vi "HEWH Channel Test Labels for RLT.vi"() -> (4 "Station A":T1, 6 "Station B":T1, 8 "Station C":T1, 10 "Station D":T1)   [LabVIEW 2011]
uses:
  Channel Label RLT.ctl
  RLT Stations.ctl
  LabelChannel.ctl
  <vilib>/Utility/file.llb/Write To Spreadsheet File (string).vi
  <vilib>/Utility/file.llb/Read From Spreadsheet File (string).vi
panel:
  out "all rows":string[][](array[string])
  in  "Read":bool
  in  "Write":bool
  in  "Initialize":bool
  in  "Complete":bool
  in  "Panel 3":T3[][](array[typedef])=[[{"Label"="TC Cond1 - IN", "Unit"=enum.""}, {"Label"="TC Cond2", "Unit"=enum.""}, {"Label"="TC Cond3", "Unit"=enum.""}, {"Label"="TC Cond4", "Unit"=enum.""}, {"Label"="TC Cond5", "Unit"=enum.""}, {"Label"="TC Cond6", "Unit"=enum.""}], [{"Label"="TC Cond7", "Unit"=enum.""}, {"Label"="TC Cond8", "Unit"=enum.""}, {"Label"="TC Cond9", "Unit"=enum.""}, {"Label"="TC Cond10", "Unit"=enum.""}, {"Label"="TC Cond11", "Unit"=enum.""}, {"Label"="TC Cond12 - OUT", "Unit"=enum.""}], [{"Label"="TC Xtra 4", "Unit"=enum.""}, {"Label"="TC Xtra 5", "Unit"=enum.""}, {"Label"="TC Xtra 6", "Unit"=enum.""}, {"Label"="TC Xtra 7", "Unit"=enum.""}, {"Label"="TC Xtra 8", "Unit"=enum.""}, {"Label"="TC Xtra 9", "Unit"=enum.""}]]
  in  "Panel 2":T3[][](array[typedef])=[[{"Label"="TC Dry/W bulb 1", "Unit"=enum.""}, {"Label"="TC Dry/W bulb 2", "Unit"=enum.""}, {"Label"="TC Dry/W bulb 3", "Unit"=enum.""}, {"Label"="TC Dry/W bulb 4", "Unit"=enum.""}, {"Label"="TC Tsuction", "Unit"=enum.""}, {"Label"="TC Tdis", "Unit"=enum.""}], [{"Label"="TC Tret", "Unit"=enum.""}, {"Label"="TC Controls 1", "Unit"=enum.""}, {"Label"="TC Controls 2", "Unit"=enum.""}, {"Label"="TC Controls 3", "Unit"=enum.""}, {"Label"="TC Controls 4", "Unit"=enum.""}, {"Label"="TC Controls 5", "Unit"=enum.""}], [{"Label"="TC Shadow T1", "Unit"=enum.""}, {"Label"="TC Shadow T2", "Unit"=enum.""}, {"Label"="TC Shadow T3", "Unit"=enum.""}, {"Label"="TC Shadow T4", "Unit"=enum.""}, {"Label"="TC Shadow T5", "Unit"=enum.""}, {"Label"="TC Shadow T6", "Unit"=enum.""}]]
  in  "Panel 1":T3[][](array[typedef])=[[{"Label"="TC Tree 1 - TOP", "Unit"=enum.""}, {"Label"="TC Tree 2", "Unit"=enum.""}, {"Label"="TC Tree 3", "Unit"=enum.""}, {"Label"="TC Tree 4", "Unit"=enum.""}, {"Label"="TC Tree 5", "Unit"=enum.""}, {"Label"="TC Tree 6 - BOT", "Unit"=enum.""}], [{"Label"="TC Shell 1", "Unit"=enum.""}, {"Label"="TC Shell 2", "Unit"=enum.""}, {"Label"="TC Shell 3", "Unit"=enum.""}, {"Label"="TC Shell 4", "Unit"=enum.""}, {"Label"="TC Evap1 - IN", "Unit"=enum.""}, {"Label"="TC Evap2", "Unit"=enum.""}], [{"Label"="TC Evap3", "Unit"=enum.""}, {"Label"="TC Evap4", "Unit"=enum.""}, {"Label"="TC Evap5 - OUT", "Unit"=enum.""}, {"Label"="TC Xtra 1", "Unit"=enum.""}, {"Label"="TC Xtra 2", "Unit"=enum.""}, {"Label"="TC Xtra 3", "Unit"=enum.""}]]
  in  "Sensor 2":T3
  # "Select Unit (A,B,C,D)  and Add Label. Using the first 10 in Panel 1 is the best."
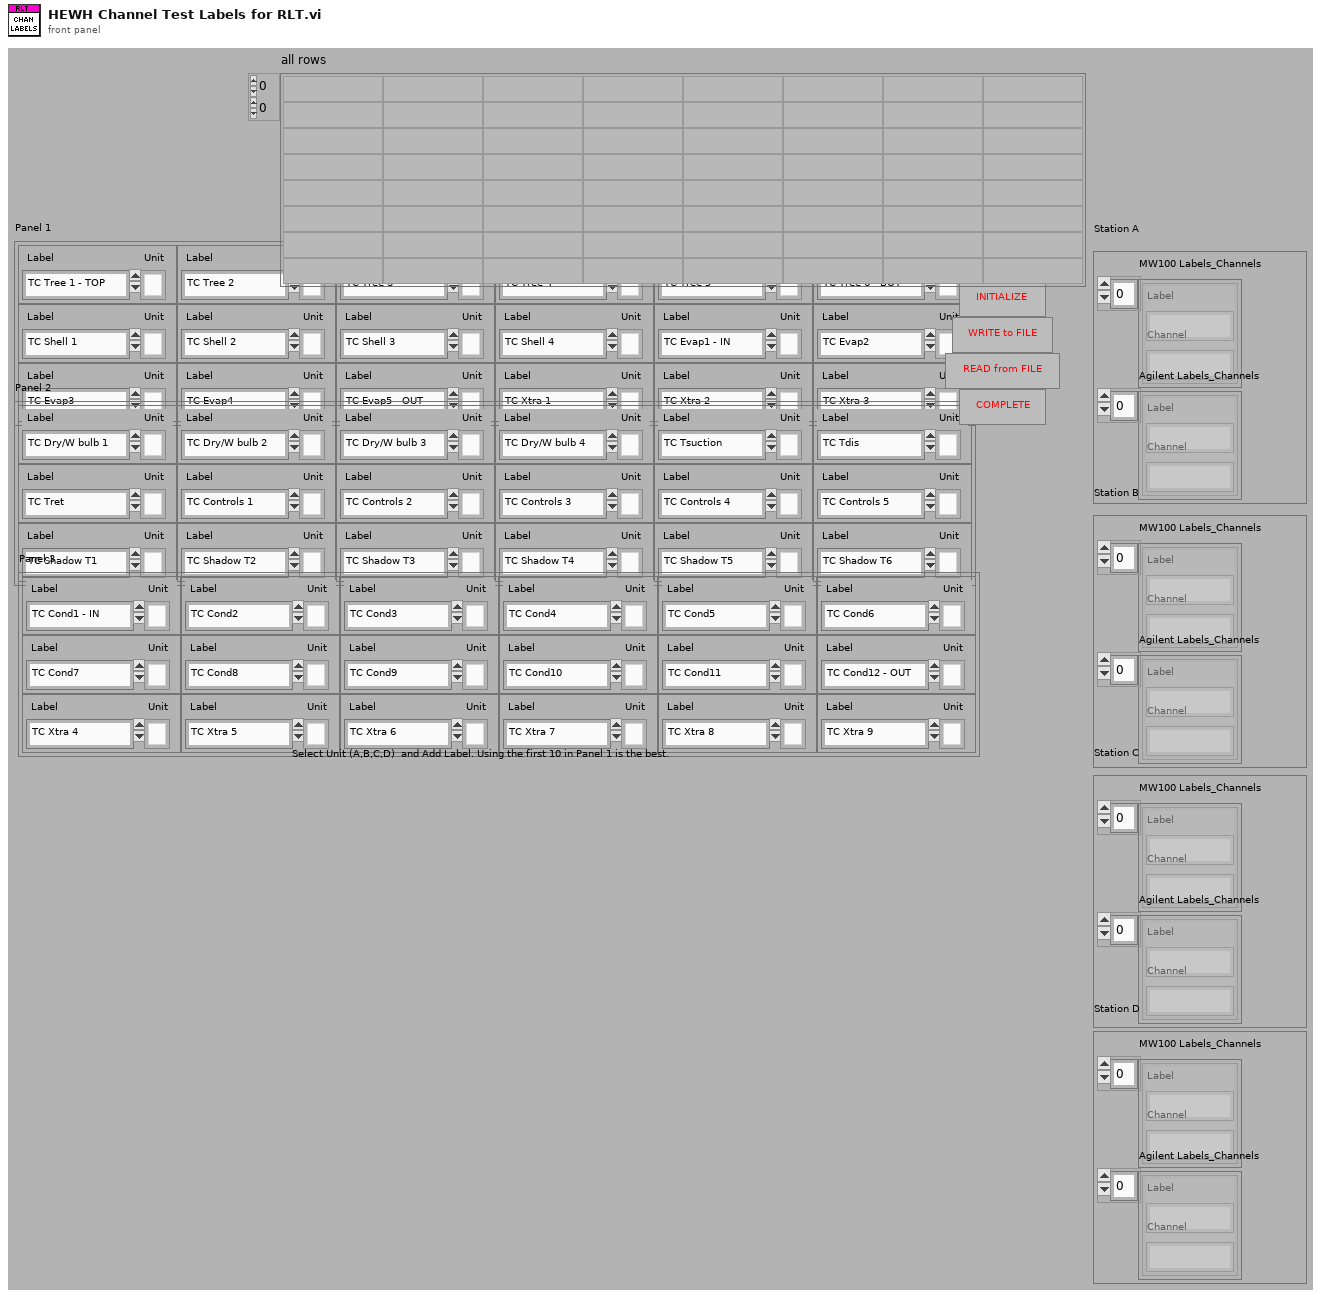
[diagram p1: front panel]
types:
  T1 = typedef "RLT Stations.ctl" = cluster{"MW100 Labels_Channels":T2[], "Agilent Labels_Channels":T2[]}
  T2 = typedef "LabelChannel.ctl" = cluster{"Label":string, "Channel":string}
  T3 = typedef "Channel Label RLT.ctl" = cluster{"Label":string, "Unit":enum16{"", "A", "B", "C", "D"}}
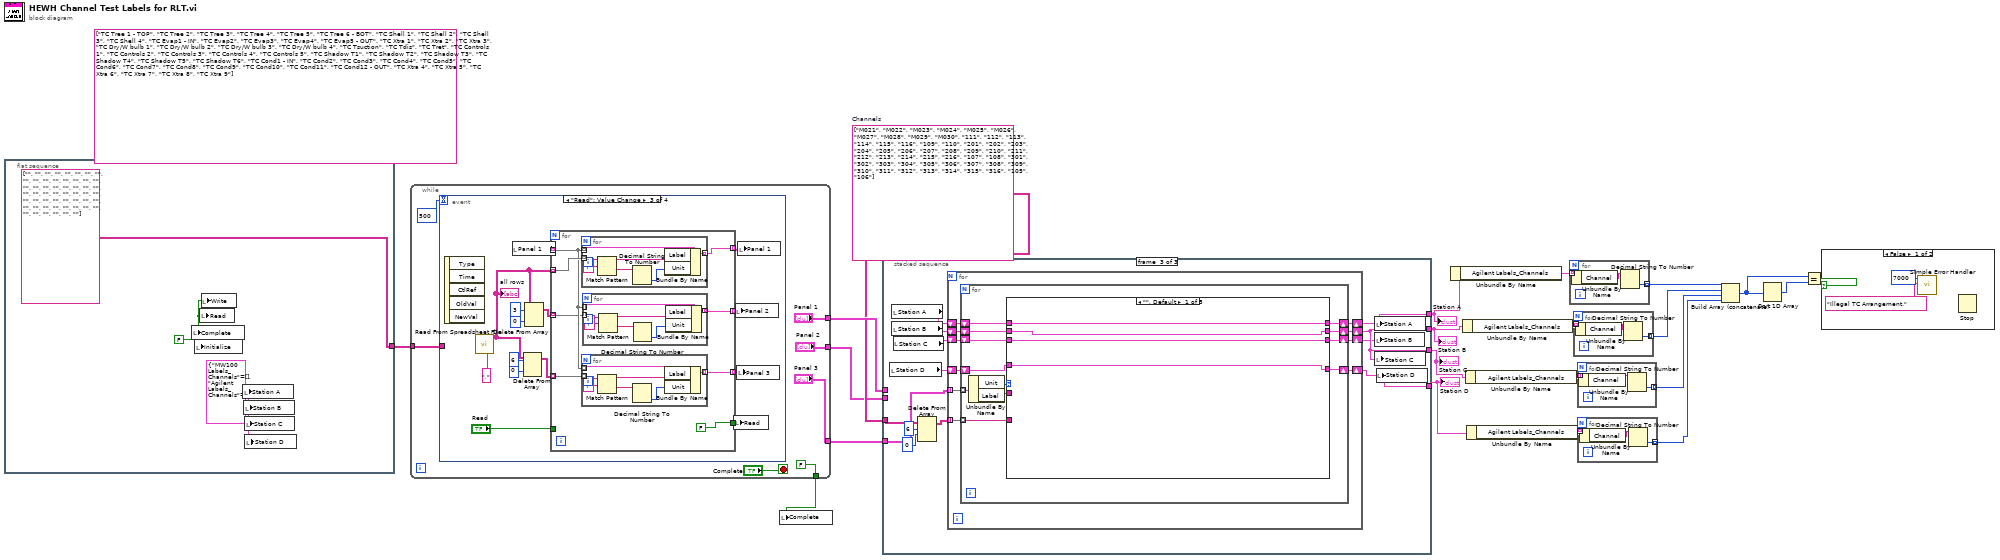
[diagram p0: block diagram]
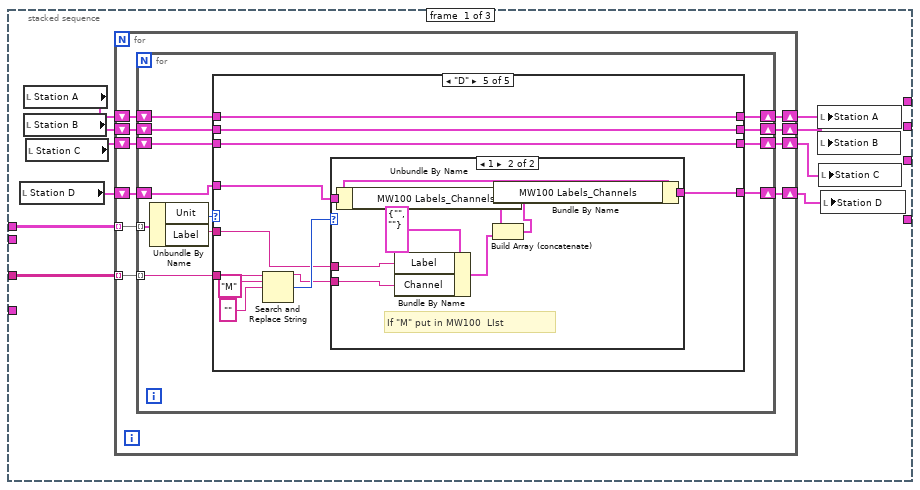
[diagram p3: hidden frame]
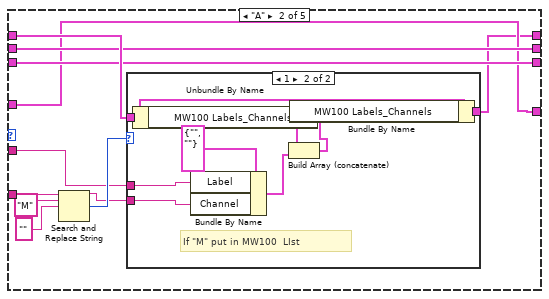
[diagram p5: hidden frame]
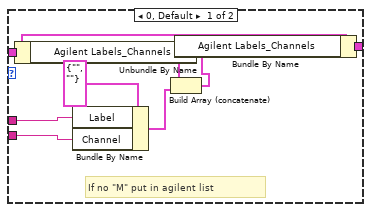
[diagram p6: hidden frame]
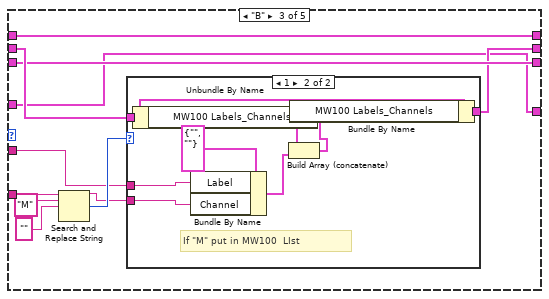
[diagram p7: hidden frame]
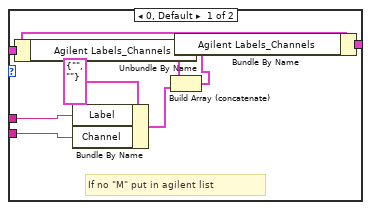
[diagram p8: hidden frame]
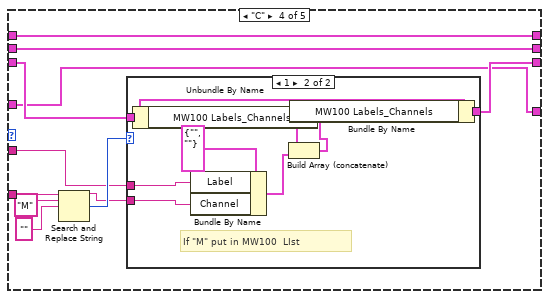
[diagram p9: hidden frame]
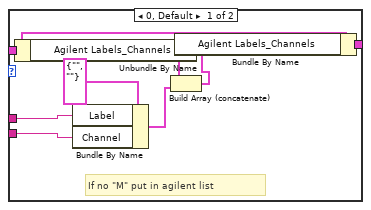
[diagram p10: hidden frame]
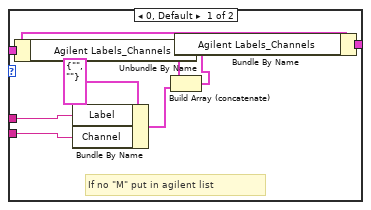
[diagram p11: hidden frame]
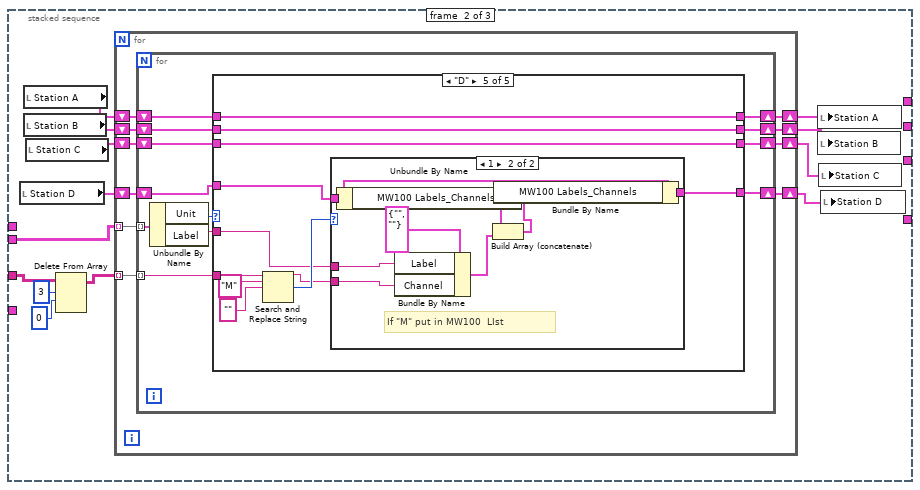
[diagram p12: hidden frame]
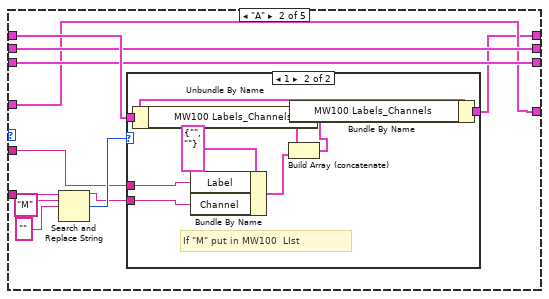
[diagram p14: hidden frame]
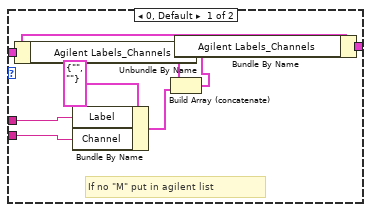
[diagram p15: hidden frame]
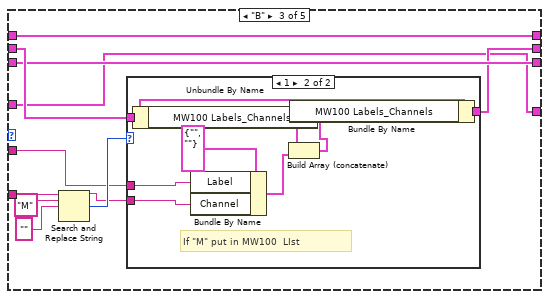
[diagram p16: hidden frame]
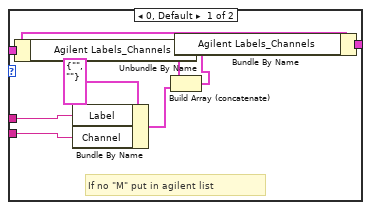
[diagram p17: hidden frame]
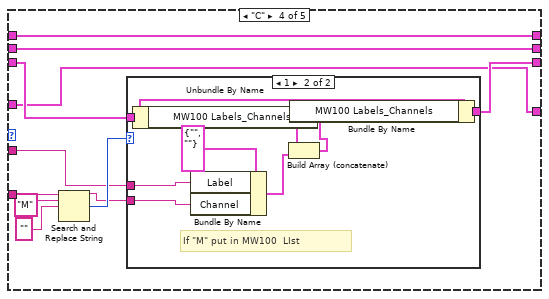
[diagram p18: hidden frame]
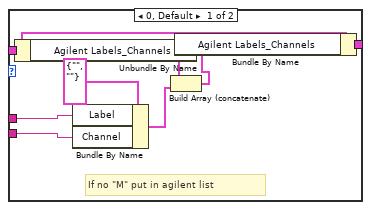
[diagram p19: hidden frame]
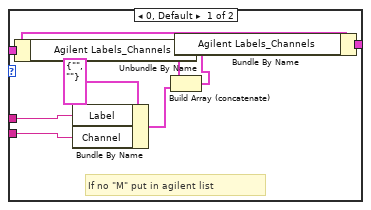
[diagram p20: hidden frame]
diagram:
  (unwired) string[][] [["TC Tree 1 - TOP", "TC Tree 2", "TC Tree 3", "TC Tree 4", "TC Tree 5", "TC Tree 6 - BOT"], ["TC Shell 1", "TC Shell 2", "TC Shell 3", "TC Shell 4", "TC Evap1 - IN", "TC Evap2"], ["TC Evap3", "TC Evap4", "TC Evap5 - OUT", "TC Xtra 1", "TC Xtra 2", "TC Xtra 3"], ["TC Dry/W bulb 1", "TC Dry/W bulb 2", "TC Dry/W bulb 3", "TC Dry/W bulb 4", "TC Tsuction", "TC Tdis"], ["TC Tret", "TC Controls 1", "TC Controls 2", "TC Controls 3", "TC Controls 4", "TC Controls 5"], ["TC Shadow T1", "TC Shadow T2", "TC Shadow T3", "TC Shadow T4", "TC Shadow T5", "TC Shadow T6"], ["TC Cond1 - IN", "TC Cond2", "TC Cond3", "TC Cond4", "TC Cond5", "TC Cond6"], ["TC Cond7", "TC Cond8", "TC Cond9", "TC Cond10", "TC Cond11", "TC Cond12 - OUT"], ["TC Xtra 4", "TC Xtra 5", "TC Xtra 6", "TC Xtra 7", "TC Xtra 8", "TC Xtra 9"]] ("Array")
  w18 = string[][] [["M021", "M022", "M023", "M024", "M025", "M026"], ["M027", "M028", "M029", "M030", "111", "112"], ["113", "114", "115", "116", "109", "110"], ["201", "202", "203", "204", "205", "206"], ["207", "208", "209", "210", "211", "212"], ["213", "214", "215", "216", "107", "108"], ["301", "302", "303", "304", "305", "306"], ["307", "308", "309", "310", "311", "312"], ["313", "314", "315", "316", "105", "106"]]  # Channels
  n1 = flat-sequence {
    tunnel: [string[][] [["", "", "", "", "", ""], ["", "", "", "", "", ""], ["", "", "", "", "", ""], ["", "", "", "", "", ""], ["", "", "", "", "", ""], ["", "", "", "", "", ""], ["", "", "", "", "", ""], ["", "", "", "", "", ""], ["", "", "", "", "", ""]] ("Array")] -> w21
    frame #0 {
      w24 = T1 {"MW100 Labels_Channels"=[], "Agilent Labels_Channels"=[]} ("Station A")
      w22 = FALSE ("Read None")
      n2 = local write "Complete"(w22) -> ()
      n3 = local write "Initialize"(w22) -> ()
      n4 = local write "Read"(w22) -> ()
      n5 = local write "Write"(w22) -> ()
      n6 = local write "Station A"(w24) -> ()
      n7 = local write "Station B"(w24) -> ()
      n8 = local write "Station C"(w24) -> ()
      n9 = local write "Station D"(w24) -> ()
    }
  }
  n10 = while {
    tunnel: w21 -> [w31]
    tunnel: ["Panel 1"] -> w19
    tunnel: ["Panel 2"] -> w17
    tunnel: ["Panel 3"] -> w16
    tunnel: [FALSE ("Read None")] -> w20
    stop <- "Complete" stop-if-true
    n11 = event shown="[2] \"Read\": Value Change" {
      selector: _ -> [_ _ _ _]
      dyn-events: _ -> [_ _ _ _]
      timeout: 500 -> [_ _ _ _]
      tunnel: w31 -> [w42 _ _ _]
      event "Initialize": Value Change {
        n12 = event-data() -> ()  [unwired: 1 in, 5 out]
        n13 = for {
          tunnel: [w45] -> w41 mode=indexing
          tunnel: w42 -> [w44] mode=indexing
          tunnel: [FALSE ("Read None")] -> w32
          n14 = for {
            tunnel: [w49] -> w45 mode=indexing
            tunnel: w44 -> [w48] mode=indexing
            n15 = Bundle By Name(cluster="Sensor 2", "Label"=w48, "Unit"=enum16{"", "A", "B", "C", "D"}."") -> (w49:T3)
          }
        }
        n16 = Delete From Array(array=w41, length=3, index (row)=0) -> (deleted portion=w35:T3[][], array with subset deleted=w36:T3[][])  [unwired: 1 in]
        n17 = local write "Initialize"(w32) -> ()
        n18 = local write "Panel 1"(w35) -> ()
        n19 = Delete From Array(array=w36, length=3, index (row)=0) -> (deleted portion=w34:T3[][], array with subset deleted=w33:T3[][])  [unwired: 1 in]
        n20 = local write "Panel 2"(w34) -> ()
        n21 = local write "Panel 3"(w33) -> ()
      }
      event "Write": Value Change {
        n22 = event-data() -> ()  [unwired: 1 in, 5 out]
        n23 = local read "Panel 3"() -> (w57:T3[][])
        n24 = local read "Panel 2"() -> (w58:T3[][])
        n25 = local read "Panel 1"() -> (w59:T3[][])
        n26 = for {
          tunnel: w59 -> [w78] mode=indexing
          tunnel: [w77] -> w54 mode=indexing
          tunnel: "Write" -> [_]
          tunnel: [FALSE ("Read")] -> w50
          n27 = for {
            tunnel: w78 -> [w84] mode=indexing
            tunnel: [w79] -> w77 mode=indexing
            n28 = Unbundle By Name(w84) -> ("Label"=w82:string, "Unit"=w83:enum16{"", "A", "B", "C", "D"})
            n29 = Number To Decimal String(number=w83) -> (decimal integer string=w80:string)  [unwired: 1 in]
            n30 = Concatenate Strings(w82, "/" ("string"), w80) -> (w79:string)
          }
        }
        n31 = for {
          tunnel: w58 -> [w69] mode=indexing
          tunnel: [w68] -> w55 mode=indexing
          n32 = for {
            tunnel: w69 -> [w75] mode=indexing
            tunnel: [w70] -> w68 mode=indexing
            n33 = Unbundle By Name(w75) -> ("Label"=w73:string, "Unit"=w74:enum16{"", "A", "B", "C", "D"})
            n34 = Number To Decimal String(number=w74) -> (decimal integer string=w71:string)  [unwired: 1 in]
            n35 = Concatenate Strings(w73, "/" ("string"), w71) -> (w70:string)
          }
        }
        n36 = for {
          tunnel: w57 -> [w61] mode=indexing
          tunnel: [w60] -> w56 mode=indexing
          n37 = for {
            tunnel: w61 -> [w67] mode=indexing
            tunnel: [w62] -> w60 mode=indexing
            n38 = Unbundle By Name(w67) -> ("Label"=w65:string, "Unit"=w66:enum16{"", "A", "B", "C", "D"})
            n39 = Number To Decimal String(number=w66) -> (decimal integer string=w63:string)  [unwired: 1 in]
            n40 = Concatenate Strings(w65, "/" ("string"), w63) -> (w62:string)
          }
        }
        n41 = Build Array (concatenate)(w54, w55, w56) -> (w53:string[][])
        n42 = local write "Write"(w50) -> ()
        n43 = call-poly <vilib>:"Write To Spreadsheet File.vi"("delimiter (\\t)"="," ("delimiter (\\t)"), "2D data"=w53) -> ()  [unwired: 6 in, 1 out]
      }
      event "Read": Value Change {
        n44 = event-data() -> ()  [unwired: 1 in, 5 out]
        n45 = call-poly <vilib>:"Read From Spreadsheet File.vi"("delimiter (\\t)"="," ("delimiter (\\t)")) -> ("all rows"=w90:string[][])  [unwired: 6 in, 4 out]
        "all rows" <- w90
        n46 = local read "Panel 1"() -> (w97:T3[][])
        n47 = Delete From Array(array=w90, length=6, index (row)=0) -> (array with subset deleted=w89:string[][])  [unwired: 1 in, 1 out]
        n48 = Delete From Array(array=w90, length=3, index (row)=0) -> (array with subset deleted=w93:string[][])  [unwired: 1 in, 1 out]
        n49 = for {
          tunnel: w97 -> [w104] mode=indexing
          tunnel: w90 -> [w106] mode=indexing
          tunnel: [w105] -> w96 mode=indexing
          tunnel: w93 -> [w103] mode=indexing
          tunnel: w89 -> [w102] mode=indexing
          tunnel: [w101] -> w88 mode=indexing
          tunnel: [w100] -> w87 mode=indexing
          tunnel: "Read" -> [_]
          tunnel: [FALSE ("Read")] -> w85
          n50 = for {
            tunnel: w104 -> [w125] mode=indexing
            tunnel: w106 -> [w127] mode=indexing
            tunnel: [w122] -> w105 mode=indexing
            n51 = Match Pattern(string=w127, regular expression="/") -> (before substring=w124:string, after substring=w123:string)  [unwired: 1 in, 2 out]
            n52 = Decimal String To Number(string=w123) -> (number=w121:i32)  [unwired: 2 in, 1 out]
            n53 = Bundle By Name(cluster=w125, "Label"=w124, "Unit"=w121) -> (w122:T3)
          }
          n54 = for {
            tunnel: w104 -> [w111] mode=indexing
            tunnel: w102 -> [w113] mode=indexing
            tunnel: [w108] -> w100 mode=indexing
            n55 = Match Pattern(string=w113, regular expression="/") -> (before substring=w110:string, after substring=w109:string)  [unwired: 1 in, 2 out]
            n56 = Decimal String To Number(string=w109) -> (number=w107:i32)  [unwired: 2 in, 1 out]
            n57 = Bundle By Name(cluster=w111, "Label"=w110, "Unit"=w107) -> (w108:T3)
          }
          n58 = for {
            tunnel: w104 -> [w118] mode=indexing
            tunnel: w103 -> [w120] mode=indexing
            tunnel: [w115] -> w101 mode=indexing
            n59 = Match Pattern(string=w120, regular expression="/") -> (before substring=w117:string, after substring=w116:string)  [unwired: 1 in, 2 out]
            n60 = Decimal String To Number(string=w116) -> (number=w114:i32)  [unwired: 2 in, 1 out]
            n61 = Bundle By Name(cluster=w118, "Label"=w117, "Unit"=w114) -> (w115:T3)
          }
        }
        n62 = local write "Read"(w85) -> ()
        n63 = local write "Panel 2"(w88) -> ()
        n64 = local write "Panel 3"(w87) -> ()
        n65 = local write "Panel 1"(w96) -> ()
      }
      event Timeout {
        n66 = event-data() -> ()  [unwired: 1 in, 2 out]
      }
    }
  }
  n67 = local write "Complete"(w20) -> ()
  n68 = stacked-sequence {
    tunnel: w19 -> [w137 _ _]
    tunnel: w18 -> [w136 w275 w419]
    tunnel: w17 -> [_ w276 _]
    tunnel: w16 -> [_ _ w427]
    tunnel: [_ _ w426] -> w8
    tunnel: [_ _ w425] -> w9
    tunnel: [_ _ w424] -> w13
    tunnel: [_ _ w423] -> w15
    frame #0 {
      n69 = local read "Station D"() -> (w128:T1)
      n70 = local read "Station A"() -> (w131:T1)
      n71 = local read "Station B"() -> (w130:T1)
      n72 = local read "Station C"() -> (w129:T1)
      n73 = for {
        tunnel: w137 -> [w147] mode=indexing
        tunnel: w136 -> [w145] mode=indexing
        shift-right: [w144] -> w135
        shift-left: w131 -> [w146]
        shift-right: [w142] -> w134
        shift-left: w130 -> [w143]
        shift-right: [w140] -> w133
        shift-left: w129 -> [w141]
        shift-right: [w138] -> w132
        shift-left: w128 -> [w139]
        n74 = for {
          tunnel: w147 -> [w159] mode=indexing
          tunnel: w145 -> [w157] mode=indexing
          shift-right: [w148] -> w144
          shift-left: w146 -> [w153]
          shift-right: [w152] -> w142
          shift-left: w143 -> [w151]
          shift-right: [w150] -> w140
          shift-left: w141 -> [w149]
          shift-right: [w154] -> w138
          shift-left: w139 -> [w155]
          n75 = Unbundle By Name(w159) -> ("Unit"=w158:enum16{"", "A", "B", "C", "D"}, "Label"=w156:string)
          n76 = case shown="\"D\"" w158 {
            tunnel: w155 -> [w160 w165 w191 w218 w251]
            tunnel: w157 -> [_ w174 w201 w228 w255]
            tunnel: w156 -> [_ w169 w196 w223 w249]
            tunnel: [w160 w165 w191 w218 w248] -> w154
            tunnel: w153 -> [w163 w168 w195 w222 w247]
            tunnel: [w162 w167 w192 w221 w246] -> w152
            tunnel: w151 -> [w162 w167 w194 w221 w246]
            tunnel: [w161 w166 w193 w219 w245] -> w150
            tunnel: w149 -> [w161 w166 w193 w220 w245]
            tunnel: [w163 w164 w195 w222 w247] -> w148
            frame "", Default {
            }
            frame "A" {
              n77 = Search and Replace String(input string=w174, search string="M", replace string="" ("replace string (\"\")")) -> (result string=w170:string, number of replacements=w171:i32)  [unwired: 5 in, 2 out]
              n78 = case shown="1" w171 {
                tunnel: w168 -> [w176 w184]
                tunnel: w170 -> [w180 w188]
                tunnel: w169 -> [w179 w187]
                tunnel: [w175 w183] -> w164
                frame 0, Default {
                  # "If no \"M\" put in agilent list"
                  n79 = Unbundle By Name(w176) -> ("Agilent Labels_Channels"=w182:T2[])
                  n80 = Bundle By Name(cluster=T2 {"Label"="", "Channel"=""} ("input cluster"), "Label"=w179, "Channel"=w180) -> (w178:T2)
                  n81 = Build Array (concatenate)(w182, w178) -> (w177:T2[])
                  n82 = Bundle By Name(cluster=w176, "Agilent Labels_Channels"=w177) -> (w175:T1)
                }
                frame 1 {
                  # "If \"M\" put in MW100  LIst"
                  n83 = Unbundle By Name(w184) -> ("MW100 Labels_Channels"=w190:T2[])
                  n84 = Bundle By Name(cluster=T2 {"Label"="", "Channel"=""} ("input cluster"), "Label"=w187, "Channel"=w188) -> (w186:T2)
                  n85 = Build Array (concatenate)(w190, w186) -> (w185:T2[])
                  n86 = Bundle By Name(cluster=w184, "MW100 Labels_Channels"=w185) -> (w183:T1)
                }
              }
            }
            frame "B" {
              n87 = Search and Replace String(input string=w201, search string="M", replace string="" ("replace string (\"\")")) -> (result string=w197:string, number of replacements=w198:i32)  [unwired: 5 in, 2 out]
              n88 = case shown="1" w198 {
                tunnel: w194 -> [w203 w211]
                tunnel: w197 -> [w207 w215]
                tunnel: w196 -> [w206 w214]
                tunnel: [w202 w210] -> w192
                frame 0, Default {
                  # "If no \"M\" put in agilent list"
                  n89 = Unbundle By Name(w203) -> ("Agilent Labels_Channels"=w209:T2[])
                  n90 = Bundle By Name(cluster=T2 {"Label"="", "Channel"=""} ("input cluster"), "Label"=w206, "Channel"=w207) -> (w205:T2)
                  n91 = Build Array (concatenate)(w209, w205) -> (w204:T2[])
                  n92 = Bundle By Name(cluster=w203, "Agilent Labels_Channels"=w204) -> (w202:T1)
                }
                frame 1 {
                  # "If \"M\" put in MW100  LIst"
                  n93 = Unbundle By Name(w211) -> ("MW100 Labels_Channels"=w217:T2[])
                  n94 = Bundle By Name(cluster=T2 {"Label"="", "Channel"=""} ("input cluster"), "Label"=w214, "Channel"=w215) -> (w213:T2)
                  n95 = Build Array (concatenate)(w217, w213) -> (w212:T2[])
                  n96 = Bundle By Name(cluster=w211, "MW100 Labels_Channels"=w212) -> (w210:T1)
                }
              }
            }
            frame "C" {
              n97 = Search and Replace String(input string=w228, search string="M", replace string="" ("replace string (\"\")")) -> (result string=w224:string, number of replacements=w225:i32)  [unwired: 5 in, 2 out]
              n98 = case shown="1" w225 {
                tunnel: w220 -> [w230 w238]
                tunnel: w224 -> [w234 w242]
                tunnel: w223 -> [w233 w241]
                tunnel: [w229 w237] -> w219
                frame 0, Default {
                  # "If no \"M\" put in agilent list"
                  n99 = Unbundle By Name(w230) -> ("Agilent Labels_Channels"=w236:T2[])
                  n100 = Bundle By Name(cluster=T2 {"Label"="", "Channel"=""} ("input cluster"), "Label"=w233, "Channel"=w234) -> (w232:T2)
                  n101 = Build Array (concatenate)(w236, w232) -> (w231:T2[])
                  n102 = Bundle By Name(cluster=w230, "Agilent Labels_Channels"=w231) -> (w229:T1)
                }
                frame 1 {
                  # "If \"M\" put in MW100  LIst"
                  n103 = Unbundle By Name(w238) -> ("MW100 Labels_Channels"=w244:T2[])
                  n104 = Bundle By Name(cluster=T2 {"Label"="", "Channel"=""} ("input cluster"), "Label"=w241, "Channel"=w242) -> (w240:T2)
                  n105 = Build Array (concatenate)(w244, w240) -> (w239:T2[])
                  n106 = Bundle By Name(cluster=w238, "MW100 Labels_Channels"=w239) -> (w237:T1)
                }
              }
            }
            frame "D" {
              n107 = Search and Replace String(input string=w255, search string="M", replace string="" ("replace string (\"\")")) -> (result string=w250:string, number of replacements=w252:i32)  [unwired: 5 in, 2 out]
              n108 = case shown="1" w252 {
                tunnel: w251 -> [w257 w265]
                tunnel: w250 -> [w261 w269]
                tunnel: w249 -> [w260 w268]
                tunnel: [w256 w264] -> w248
                frame 0, Default {
                  # "If no \"M\" put in agilent list"
                  n109 = Unbundle By Name(w257) -> ("Agilent Labels_Channels"=w263:T2[])
                  n110 = Bundle By Name(cluster=T2 {"Label"="", "Channel"=""} ("input cluster"), "Label"=w260, "Channel"=w261) -> (w259:T2)
                  n111 = Build Array (concatenate)(w263, w259) -> (w258:T2[])
                  n112 = Bundle By Name(cluster=w257, "Agilent Labels_Channels"=w258) -> (w256:T1)
                }
                frame 1 {
                  # "If \"M\" put in MW100  LIst"
                  n113 = Unbundle By Name(w265) -> ("MW100 Labels_Channels"=w271:T2[])
                  n114 = Bundle By Name(cluster=T2 {"Label"="", "Channel"=""} ("input cluster"), "Label"=w268, "Channel"=w269) -> (w267:T2)
                  n115 = Build Array (concatenate)(w271, w267) -> (w266:T2[])
                  n116 = Bundle By Name(cluster=w265, "MW100 Labels_Channels"=w266) -> (w264:T1)
                }
              }
            }
          }
        }
      }
      n117 = local write "Station A"(w135) -> ()
      n118 = local write "Station B"(w134) -> ()
      n119 = local write "Station C"(w133) -> ()
      n120 = local write "Station D"(w132) -> ()
    }
    frame #1 {
      n121 = local read "Station D"() -> (w277:T1)
      n122 = local read "Station A"() -> (w280:T1)
      n123 = local read "Station B"() -> (w279:T1)
      n124 = local read "Station C"() -> (w278:T1)
      n125 = Delete From Array(array=w275, length=3, index (row)=0) -> (array with subset deleted=w272:string[][])  [unwired: 1 in, 1 out]
      n126 = for {
        tunnel: w276 -> [w294] mode=indexing
        tunnel: w272 -> [w292] mode=indexing
        shift-right: [w291] -> w284
        shift-left: w280 -> [w293]
        shift-right: [w289] -> w283
        shift-left: w279 -> [w290]
        shift-right: [w287] -> w282
        shift-left: w278 -> [w288]
        shift-right: [w285] -> w281
        shift-left: w277 -> [w286]
        n127 = for {
          tunnel: w294 -> [w306] mode=indexing
          tunnel: w292 -> [w304] mode=indexing
          shift-right: [w295] -> w291
          shift-left: w293 -> [w300]
          shift-right: [w299] -> w289
          shift-left: w290 -> [w298]
          shift-right: [w297] -> w287
          shift-left: w288 -> [w296]
          shift-right: [w301] -> w285
          shift-left: w286 -> [w302]
          n128 = Unbundle By Name(w306) -> ("Unit"=w305:enum16{"", "A", "B", "C", "D"}, "Label"=w303:string)
          n129 = case shown="\"D\"" w305 {
            tunnel: w302 -> [w307 w312 w338 w365 w398]
            tunnel: w304 -> [_ w321 w348 w375 w402]
            tunnel: w303 -> [_ w316 w343 w370 w396]
            tunnel: [w307 w312 w338 w365 w395] -> w301
            tunnel: w300 -> [w310 w315 w342 w369 w394]
            tunnel: [w309 w314 w339 w368 w393] -> w299
            tunnel: w298 -> [w309 w314 w341 w368 w393]
            tunnel: [w308 w313 w340 w366 w392] -> w297
            tunnel: w296 -> [w308 w313 w340 w367 w392]
            tunnel: [w310 w311 w342 w369 w394] -> w295
            frame "", Default {
            }
            frame "A" {
              n130 = Search and Replace String(input string=w321, search string="M", replace string="" ("replace string (\"\")")) -> (result string=w317:string, number of replacements=w318:i32)  [unwired: 5 in, 2 out]
              n131 = case shown="1" w318 {
                tunnel: w315 -> [w323 w331]
                tunnel: w317 -> [w327 w335]
                tunnel: w316 -> [w326 w334]
                tunnel: [w322 w330] -> w311
                frame 0, Default {
                  # "If no \"M\" put in agilent list"
                  n132 = Unbundle By Name(w323) -> ("Agilent Labels_Channels"=w329:T2[])
                  n133 = Bundle By Name(cluster=T2 {"Label"="", "Channel"=""} ("input cluster"), "Label"=w326, "Channel"=w327) -> (w325:T2)
                  n134 = Build Array (concatenate)(w329, w325) -> (w324:T2[])
                  n135 = Bundle By Name(cluster=w323, "Agilent Labels_Channels"=w324) -> (w322:T1)
                }
                frame 1 {
                  # "If \"M\" put in MW100  LIst"
                  n136 = Unbundle By Name(w331) -> ("MW100 Labels_Channels"=w337:T2[])
                  n137 = Bundle By Name(cluster=T2 {"Label"="", "Channel"=""} ("input cluster"), "Label"=w334, "Channel"=w335) -> (w333:T2)
                  n138 = Build Array (concatenate)(w337, w333) -> (w332:T2[])
                  n139 = Bundle By Name(cluster=w331, "MW100 Labels_Channels"=w332) -> (w330:T1)
                }
              }
            }
            frame "B" {
              n140 = Search and Replace String(input string=w348, search string="M", replace string="" ("replace string (\"\")")) -> (result string=w344:string, number of replacements=w345:i32)  [unwired: 5 in, 2 out]
              n141 = case shown="1" w345 {
                tunnel: w341 -> [w350 w358]
                tunnel: w344 -> [w354 w362]
                tunnel: w343 -> [w353 w361]
                tunnel: [w349 w357] -> w339
                frame 0, Default {
                  # "If no \"M\" put in agilent list"
                  n142 = Unbundle By Name(w350) -> ("Agilent Labels_Channels"=w356:T2[])
                  n143 = Bundle By Name(cluster=T2 {"Label"="", "Channel"=""} ("input cluster"), "Label"=w353, "Channel"=w354) -> (w352:T2)
                  n144 = Build Array (concatenate)(w356, w352) -> (w351:T2[])
                  n145 = Bundle By Name(cluster=w350, "Agilent Labels_Channels"=w351) -> (w349:T1)
                }
                frame 1 {
                  # "If \"M\" put in MW100  LIst"
                  n146 = Unbundle By Name(w358) -> ("MW100 Labels_Channels"=w364:T2[])
                  n147 = Bundle By Name(cluster=T2 {"Label"="", "Channel"=""} ("input cluster"), "Label"=w361, "Channel"=w362) -> (w360:T2)
                  n148 = Build Array (concatenate)(w364, w360) -> (w359:T2[])
                  n149 = Bundle By Name(cluster=w358, "MW100 Labels_Channels"=w359) -> (w357:T1)
                }
              }
            }
            frame "C" {
              n150 = Search and Replace String(input string=w375, search string="M", replace string="" ("replace string (\"\")")) -> (result string=w371:string, number of replacements=w372:i32)  [unwired: 5 in, 2 out]
              n151 = case shown="1" w372 {
                tunnel: w367 -> [w377 w385]
                tunnel: w371 -> [w381 w389]
                tunnel: w370 -> [w380 w388]
                tunnel: [w376 w384] -> w366
                frame 0, Default {
                  # "If no \"M\" put in agilent list"
                  n152 = Unbundle By Name(w377) -> ("Agilent Labels_Channels"=w383:T2[])
                  n153 = Bundle By Name(cluster=T2 {"Label"="", "Channel"=""} ("input cluster"), "Label"=w380, "Channel"=w381) -> (w379:T2)
                  n154 = Build Array (concatenate)(w383, w379) -> (w378:T2[])
                  n155 = Bundle By Name(cluster=w377, "Agilent Labels_Channels"=w378) -> (w376:T1)
                }
                frame 1 {
                  # "If \"M\" put in MW100  LIst"
                  n156 = Unbundle By Name(w385) -> ("MW100 Labels_Channels"=w391:T2[])
                  n157 = Bundle By Name(cluster=T2 {"Label"="", "Channel"=""} ("input cluster"), "Label"=w388, "Channel"=w389) -> (w387:T2)
                  n158 = Build Array (concatenate)(w391, w387) -> (w386:T2[])
                  n159 = Bundle By Name(cluster=w385, "MW100 Labels_Channels"=w386) -> (w384:T1)
                }
              }
            }
            frame "D" {
              n160 = Search and Replace String(input string=w402, search string="M", replace string="" ("replace string (\"\")")) -> (result string=w397:string, number of replacements=w399:i32)  [unwired: 5 in, 2 out]
              n161 = case shown="1" w399 {
                tunnel: w398 -> [w404 w412]
                tunnel: w397 -> [w408 w416]
                tunnel: w396 -> [w407 w415]
                tunnel: [w403 w411] -> w395
                frame 0, Default {
                  # "If no \"M\" put in agilent list"
                  n162 = Unbundle By Name(w404) -> ("Agilent Labels_Channels"=w410:T2[])
                  n163 = Bundle By Name(cluster=T2 {"Label"="", "Channel"=""} ("input cluster"), "Label"=w407, "Channel"=w408) -> (w406:T2)
                  n164 = Build Array (concatenate)(w410, w406) -> (w405:T2[])
                  n165 = Bundle By Name(cluster=w404, "Agilent Labels_Channels"=w405) -> (w403:T1)
                }
                frame 1 {
                  # "If \"M\" put in MW100  LIst"
                  n166 = Unbundle By Name(w412) -> ("MW100 Labels_Channels"=w418:T2[])
                  n167 = Bundle By Name(cluster=T2 {"Label"="", "Channel"=""} ("input cluster"), "Label"=w415, "Channel"=w416) -> (w414:T2)
                  n168 = Build Array (concatenate)(w418, w414) -> (w413:T2[])
                  n169 = Bundle By Name(cluster=w412, "MW100 Labels_Channels"=w413) -> (w411:T1)
                }
              }
            }
          }
        }
      }
      n170 = local write "Station A"(w284) -> ()
      n171 = local write "Station B"(w283) -> ()
      n172 = local write "Station C"(w282) -> ()
      n173 = local write "Station D"(w281) -> ()
    }
    frame #2 {
      n174 = local read "Station D"() -> (w428:T1)
      n175 = local read "Station A"() -> (w431:T1)
      n176 = local read "Station B"() -> (w430:T1)
      n177 = local read "Station C"() -> (w429:T1)
      n178 = Delete From Array(array=w419, length=6, index (row)=0) -> (array with subset deleted=w420:string[][])  [unwired: 1 in, 1 out]
      n179 = for {
        tunnel: w427 -> [w441] mode=indexing
        tunnel: w420 -> [w439] mode=indexing
        shift-right: [w438] -> w423
        shift-left: w431 -> [w440]
        shift-right: [w436] -> w424
        shift-left: w430 -> [w437]
        shift-right: [w434] -> w425
        shift-left: w429 -> [w435]
        shift-right: [w432] -> w426
        shift-left: w428 -> [w433]
        n180 = for {
          tunnel: w441 -> [w453] mode=indexing
          tunnel: w439 -> [w451] mode=indexing
          shift-right: [w442] -> w438
          shift-left: w440 -> [w447]
          shift-right: [w446] -> w436
          shift-left: w437 -> [w445]
          shift-right: [w444] -> w434
          shift-left: w435 -> [w443]
          shift-right: [w448] -> w432
          shift-left: w433 -> [w449]
          n181 = Unbundle By Name(w453) -> ("Unit"=w452:enum16{"", "A", "B", "C", "D"}, "Label"=w450:string)
          n182 = case shown="\"\", Default" w452 {
            tunnel: w449 -> [w454 w459 w485 w512 w545]
            tunnel: w451 -> [_ w468 w495 w522 w549]
            tunnel: w450 -> [_ w463 w490 w517 w543]
            tunnel: [w454 w459 w485 w512 w542] -> w448
            tunnel: w447 -> [w457 w462 w489 w516 w541]
            tunnel: [w456 w461 w486 w515 w540] -> w446
            tunnel: w445 -> [w456 w461 w488 w515 w540]
            tunnel: [w455 w460 w487 w513 w539] -> w444
            tunnel: w443 -> [w455 w460 w487 w514 w539]
            tunnel: [w457 w458 w489 w516 w541] -> w442
            frame "", Default {
            }
            frame "A" {
              n183 = Search and Replace String(input string=w468, search string="M", replace string="" ("replace string (\"\")")) -> (result string=w464:string, number of replacements=w465:i32)  [unwired: 5 in, 2 out]
              n184 = case shown="1" w465 {
                tunnel: w462 -> [w470 w478]
                tunnel: w464 -> [w474 w482]
                tunnel: w463 -> [w473 w481]
                tunnel: [w469 w477] -> w458
                frame 0, Default {
                  # "If no \"M\" put in agilent list"
                  n185 = Unbundle By Name(w470) -> ("Agilent Labels_Channels"=w476:T2[])
                  n186 = Bundle By Name(cluster=T2 {"Label"="", "Channel"=""} ("input cluster"), "Label"=w473, "Channel"=w474) -> (w472:T2)
                  n187 = Build Array (concatenate)(w476, w472) -> (w471:T2[])
                  n188 = Bundle By Name(cluster=w470, "Agilent Labels_Channels"=w471) -> (w469:T1)
                }
                frame 1 {
                  # "If \"M\" put in MW100  LIst"
                  n189 = Unbundle By Name(w478) -> ("MW100 Labels_Channels"=w484:T2[])
                  n190 = Bundle By Name(cluster=T2 {"Label"="", "Channel"=""} ("input cluster"), "Label"=w481, "Channel"=w482) -> (w480:T2)
                  n191 = Build Array (concatenate)(w484, w480) -> (w479:T2[])
                  n192 = Bundle By Name(cluster=w478, "MW100 Labels_Channels"=w479) -> (w477:T1)
                }
              }
            }
            frame "B" {
              n193 = Search and Replace String(input string=w495, search string="M", replace string="" ("replace string (\"\")")) -> (result string=w491:string, number of replacements=w492:i32)  [unwired: 5 in, 2 out]
              n194 = case shown="1" w492 {
                tunnel: w488 -> [w497 w505]
                tunnel: w491 -> [w501 w509]
                tunnel: w490 -> [w500 w508]
                tunnel: [w496 w504] -> w486
                frame 0, Default {
                  # "If no \"M\" put in agilent list"
                  n195 = Unbundle By Name(w497) -> ("Agilent Labels_Channels"=w503:T2[])
                  n196 = Bundle By Name(cluster=T2 {"Label"="", "Channel"=""} ("input cluster"), "Label"=w500, "Channel"=w501) -> (w499:T2)
                  n197 = Build Array (concatenate)(w503, w499) -> (w498:T2[])
                  n198 = Bundle By Name(cluster=w497, "Agilent Labels_Channels"=w498) -> (w496:T1)
                }
                frame 1 {
                  # "If \"M\" put in MW100  LIst"
                  n199 = Unbundle By Name(w505) -> ("MW100 Labels_Channels"=w511:T2[])
                  n200 = Bundle By Name(cluster=T2 {"Label"="", "Channel"=""} ("input cluster"), "Label"=w508, "Channel"=w509) -> (w507:T2)
                  n201 = Build Array (concatenate)(w511, w507) -> (w506:T2[])
                  n202 = Bundle By Name(cluster=w505, "MW100 Labels_Channels"=w506) -> (w504:T1)
                }
              }
            }
            frame "C" {
              n203 = Search and Replace String(input string=w522, search string="M", replace string="" ("replace string (\"\")")) -> (result string=w518:string, number of replacements=w519:i32)  [unwired: 5 in, 2 out]
              n204 = case shown="1" w519 {
                tunnel: w514 -> [w524 w532]
                tunnel: w518 -> [w528 w536]
                tunnel: w517 -> [w527 w535]
                tunnel: [w523 w531] -> w513
                frame 0, Default {
                  # "If no \"M\" put in agilent list"
                  n205 = Unbundle By Name(w524) -> ("Agilent Labels_Channels"=w530:T2[])
                  n206 = Bundle By Name(cluster=T2 {"Label"="", "Channel"=""} ("input cluster"), "Label"=w527, "Channel"=w528) -> (w526:T2)
                  n207 = Build Array (concatenate)(w530, w526) -> (w525:T2[])
                  n208 = Bundle By Name(cluster=w524, "Agilent Labels_Channels"=w525) -> (w523:T1)
                }
                frame 1 {
                  # "If \"M\" put in MW100  LIst"
                  n209 = Unbundle By Name(w532) -> ("MW100 Labels_Channels"=w538:T2[])
                  n210 = Bundle By Name(cluster=T2 {"Label"="", "Channel"=""} ("input cluster"), "Label"=w535, "Channel"=w536) -> (w534:T2)
                  n211 = Build Array (concatenate)(w538, w534) -> (w533:T2[])
                  n212 = Bundle By Name(cluster=w532, "MW100 Labels_Channels"=w533) -> (w531:T1)
                }
              }
            }
            frame "D" {
              n213 = Search and Replace String(input string=w549, search string="M", replace string="" ("replace string (\"\")")) -> (result string=w544:string, number of replacements=w546:i32)  [unwired: 5 in, 2 out]
              n214 = case shown="0, Default" w546 {
                tunnel: w545 -> [w551 w559]
                tunnel: w544 -> [w555 w563]
                tunnel: w543 -> [w554 w562]
                tunnel: [w550 w558] -> w542
                frame 0, Default {
                  # "If no \"M\" put in agilent list"
                  n215 = Unbundle By Name(w551) -> ("Agilent Labels_Channels"=w557:T2[])
                  n216 = Bundle By Name(cluster=T2 {"Label"="", "Channel"=""} ("input cluster"), "Label"=w554, "Channel"=w555) -> (w553:T2)
                  n217 = Build Array (concatenate)(w557, w553) -> (w552:T2[])
                  n218 = Bundle By Name(cluster=w551, "Agilent Labels_Channels"=w552) -> (w550:T1)
                }
                frame 1 {
                  # "If \"M\" put in MW100  LIst"
                  n219 = Unbundle By Name(w559) -> ("MW100 Labels_Channels"=w565:T2[])
                  n220 = Bundle By Name(cluster=T2 {"Label"="", "Channel"=""} ("input cluster"), "Label"=w562, "Channel"=w563) -> (w561:T2)
                  n221 = Build Array (concatenate)(w565, w561) -> (w560:T2[])
                  n222 = Bundle By Name(cluster=w559, "MW100 Labels_Channels"=w560) -> (w558:T1)
                }
              }
            }
          }
        }
      }
      n223 = local write "Station A"(w423) -> ()
      n224 = local write "Station B"(w424) -> ()
      n225 = local write "Station C"(w425) -> ()
      n226 = local write "Station D"(w426) -> ()
    }
  }
  "Station C" <- w9
  "Station A" <- w15
  "Station B" <- w13
  "Station D" <- w8
  n227 = Unbundle By Name(w15) -> ("Agilent Labels_Channels"=w14:T2[])
  n228 = Unbundle By Name(w13) -> ("Agilent Labels_Channels"=w12:T2[])
  n229 = Unbundle By Name(w9) -> ("Agilent Labels_Channels"=w11:T2[])
  n230 = Unbundle By Name(w8) -> ("Agilent Labels_Channels"=w10:T2[])
  n231 = for {
    tunnel: w14 -> [w568] mode=indexing
    tunnel: [w566] -> w4 mode=indexing
    n232 = Unbundle By Name(w568) -> ("Channel"=w567:string)
    n233 = Decimal String To Number(string=w567) -> (number=w566:i32)  [unwired: 2 in, 1 out]
  }
  n234 = for {
    tunnel: w12 -> [w571] mode=indexing
    tunnel: [w569] -> w5 mode=indexing
    n235 = Unbundle By Name(w571) -> ("Channel"=w570:string)
    n236 = Decimal String To Number(string=w570) -> (number=w569:i32)  [unwired: 2 in, 1 out]
  }
  n237 = for {
    tunnel: w11 -> [w574] mode=indexing
    tunnel: [w572] -> w6 mode=indexing
    n238 = Unbundle By Name(w574) -> ("Channel"=w573:string)
    n239 = Decimal String To Number(string=w573) -> (number=w572:i32)  [unwired: 2 in, 1 out]
  }
  n240 = for {
    tunnel: w10 -> [w577] mode=indexing
    tunnel: [w575] -> w7 mode=indexing
    n241 = Unbundle By Name(w577) -> ("Channel"=w576:string)
    n242 = Decimal String To Number(string=w576) -> (number=w575:i32)  [unwired: 2 in, 1 out]
  }
  n243 = Build Array (concatenate)(w4, w5, w6, w7) -> (w2:i32[])
  n244 = Sort 1D Array(array=w2) -> (sorted array=w3:i32[])
  n245 = Equal?(x=w2, y=w3) -> (x = y?=w1:bool)
  n246 = case shown="False" w1 {
    frame False {
      n247 = call <vilib>:"Simple Error Handler.vi"("error code (no error:0)"=7000, "error source (\" \")"="Illegal TC Arrangement." ("error source (\" \")")) -> ()  [unwired: 3 in, 5 out]
      n248 = Stop() -> ()  [unwired: 1 in]
    }
    frame True {
    }
  }
